vi "find_e.vi"(4 "subtract":dbl, 8 "delta thresh":dbl=2.0, 9 "square thresh":i32=2, 10 "e-size":u8, 11 "input array":dbl[][](array[numeric])) -> (3 "locations":dbl[][](array[numeric]))   [LabVIEW 2015]
uses:
  <vilib>/Analysis/_algsub.llb/Real Vector Norm.vi
  <vilib>/Analysis/baseanly.llb/Mean (DBL).vi
  <vilib>/Analysis/NI_AALPro.lvlib
  <vilib>/Analysis/NI_AALBase.lvlib
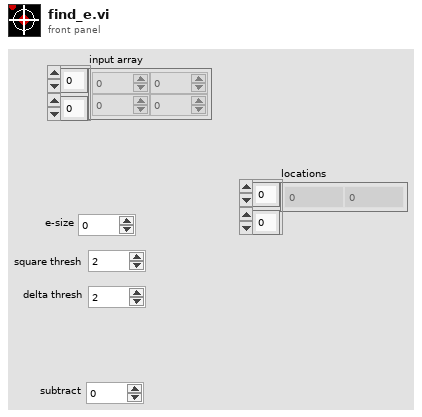
[diagram p1: front panel]
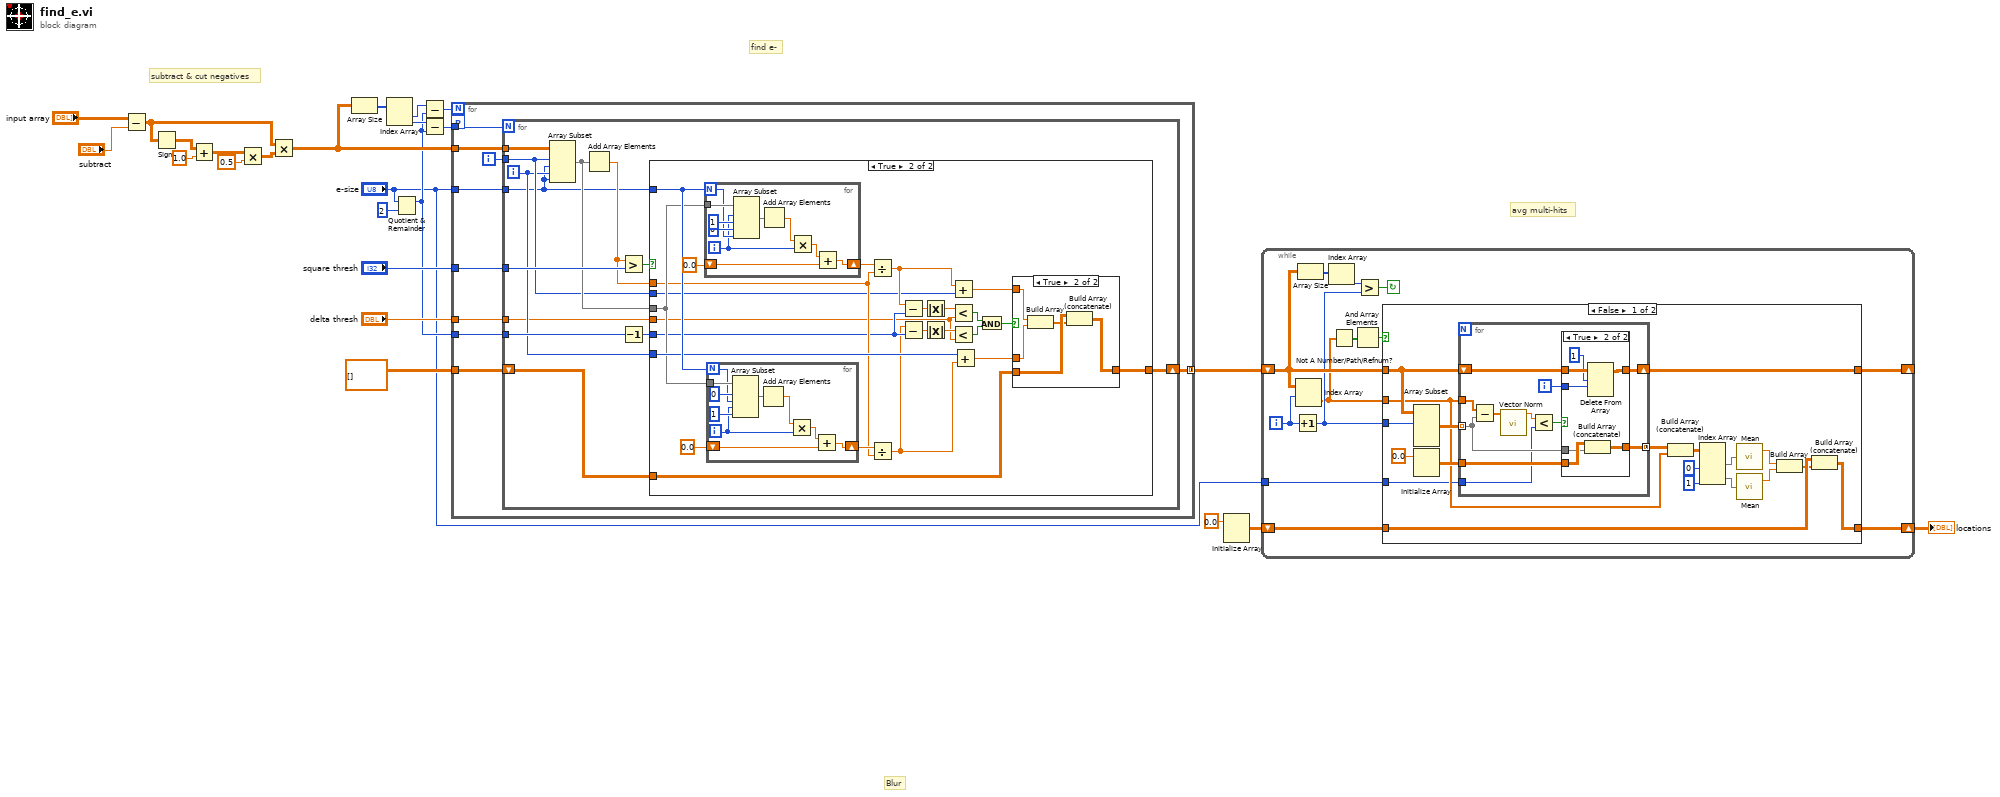
[diagram p0: block diagram]
diagram:
  # "subtract & cut negatives"
  # "avg multi-hits"
  # "find e-"
  # "Blur"
  n1 = Subtract(x="input array", y="subtract") -> (x-y=w10:dbl[][])
  n2 = Sign(1:w10) -> (0:w5:dbl[][])
  n3 = Add(x=w5, y=1.0) -> (x+y=w7:dbl[][])
  n4 = Multiply(x=w7, y=0.5) -> (x*y=w9:dbl[][])
  n5 = Multiply(x=w10, y=w9) -> (x*y=w19:dbl[][])
  n6 = Array Size(array=w19) -> (size(s)=w18:i32[])
  n7 = Index Array(array=w18) -> (element #1=w17:i32, element #2=w16:i32)  [unwired: 2 in]
  n8 = Quotient & Remainder(x="e-size", y=u8 2) -> (x-y*floor(x/y)=w3:u8)  [unwired: 1 out]
  n9 = Subtract(x=w17, y=w3) -> (x-y=w15:i32)
  n10 = Subtract(x=w16, y=w3) -> (x-y=w14:i32)
  n11 = for {
    N: w15 -> [_]
    tunnel: w19 -> [w33]
    tunnel: w14 -> [w32]
    tunnel: "e-size" -> [w30]
    tunnel: w3 -> [w29]
    tunnel: "square thresh" -> [w26]
    workers-P: _ -> [_]
    tunnel: dbl[][] [] -> [w28]
    tunnel: [w27] -> w24 mode=concatenating
    tunnel: "delta thresh" -> [w25]
    i -> [w31]
    n12 = for {
      N: w32 -> [_]
      tunnel: w33 -> [w46]
      tunnel: w31 -> [w38]
      tunnel: w30 -> [w34]
      tunnel: w29 -> [w42]
      shift-right: [w44] -> w27
      shift-left: w28 -> [w45]
      tunnel: w26 -> [w41]
      tunnel: w25 -> [w35]
      i -> [w37]
      n13 = Array Subset(array=w46, index (row)=w38, length (row)=w34, index (col)=w37, length (col)=w34) -> (w39:dbl[][])
      n14 = Add Array Elements(numeric array=w39) -> (sum=w36:dbl)
      n15 = Greater?(x=w36, y=w41) -> (0:w40:bool)
      n16 = Decrement(x=w42) -> (x-1=w43:u8)
      n17 = case shown="True" w40 {
        tunnel: w45 -> [w47 w69]
        tunnel: [w47 w68] -> w44
        tunnel: w43 -> [_ w59]
        tunnel: w34 -> [_ w67]
        tunnel: w38 -> [_ w49]
        tunnel: w37 -> [_ w64]
        tunnel: w39 -> [_ w63]
        tunnel: w36 -> [_ w60]
        tunnel: w35 -> [_ w54]
        frame False {
        }
        frame True {
          n18 = for {
            N: w67 -> [w94]
            tunnel: w63 -> [w97]
            shift-right: [w88] -> w62
            shift-left: 0.0 -> [w89]
            i -> [w91]
            n19 = Array Subset(array=w97, index (row)=w91, length (row)=1 ("Länge"), index (col)=0 ("Index"), length (col)=w94) -> (w93:dbl[][])
            n20 = Add Array Elements(numeric array=w93) -> (sum=w92:dbl)
            n21 = Multiply(x=w92, y=w91) -> (x*y=w90:dbl)
            n22 = Add(x=w90, y=w89) -> (x+y=w88:dbl)
          }
          n23 = for {
            N: w67 -> [w80]
            tunnel: w63 -> [w87]
            shift-right: [w82] -> w61
            shift-left: 0.0 -> [w83]
            i -> [w78]
            n24 = Array Subset(array=w87, index (row)=0 ("Index"), length (row)=w80, index (col)=w78, length (col)=1 ("Länge")) -> (w86:dbl[][])
            n25 = Add Array Elements(numeric array=w86) -> (sum=w85:dbl)
            n26 = Multiply(x=w85, y=w78) -> (x*y=w84:dbl)
            n27 = Add(x=w84, y=w83) -> (x+y=w82:dbl)
          }
          n28 = Divide(x=w62, y=w60) -> (x/y=w50:dbl)
          n29 = Divide(x=w61, y=w60) -> (x/y=w51:dbl)
          n30 = Subtract(x=w50, y=w59) -> (x-y=w58:dbl)
          n31 = Subtract(x=w51, y=w59) -> (x-y=w57:dbl)
          n32 = Absolute Value(x=w58) -> (abs(x)=w56:dbl)
          n33 = Absolute Value(x=w57) -> (abs(x)=w55:dbl)
          n34 = Add(x=w50, y=w49) -> (x+y=w66:dbl)
          n35 = Less?(x=w56, y=w54) -> (x < y?=w52:bool)
          n36 = Less?(x=w55, y=w54) -> (x < y?=w53:bool)
          n37 = Add(x=w64, y=w51) -> (x+y=w65:dbl)
          n38 = And(x=w52, y=w53) -> (x .and. y?=w70:bool)
          n39 = case shown="True" w70 {
            tunnel: w66 -> [_ w76]
            tunnel: w65 -> [_ w75]
            tunnel: w69 -> [w72 w77]
            tunnel: [w72 w73] -> w68
            frame False {
            }
            frame True {
              n40 = Build Array(w76, w75) -> (w74:dbl[])
              n41 = Build Array (concatenate)(w77, w74) -> (w73:dbl[][])
            }
          }
        }
      }
    }
  }
  n42 = Initialize Array(0.0 ("element")) -> (w22:dbl[][])  [unwired: 2 in]
  n43 = while {
    shift-right: [w108] -> _
    shift-left: w24 -> [w107]
    shift-right: [w109] -> w21
    shift-left: w22 -> [w110]
    tunnel: "e-size" -> [w98]
    i -> [w105]
    stop <- w102 continue-if-true
    n44 = Increment(x=w105) -> (x+1=w103:i32)
    n45 = Index Array(array=w107, index (row)=w105) -> (element=w101:dbl[])  [unwired: 1 in]
    n46 = Array Size(array=w107) -> (size(s)=w106:i32[])
    n47 = Index Array(array=w106) -> (element=w104:i32)  [unwired: 1 in]
    n48 = Not A Number/Path/Refnum?(number/path/refnum=w101) -> (NaN/Path/Refnum?=w100:bool[])
    n49 = And Array Elements(Boolean array=w100) -> (logical AND=w99:bool)
    n50 = Greater?(x=w104, y=w103) -> (0:w102:bool)
    n51 = case shown="False" w99 {
      tunnel: w110 -> [w129 w150]
      tunnel: [w128 w150] -> w109
      tunnel: [w127 w151] -> w108
      tunnel: w107 -> [w116 w151]
      tunnel: w103 -> [w115 _]
      tunnel: w101 -> [w112 _]
      tunnel: w98 -> [w111 _]
      frame False {
        n52 = Array Subset(array=w116, index (row)=w115) -> (w126:dbl[][])  [unwired: 3 in]
        n53 = Initialize Array(0.0 ("element")) -> (w124:dbl[][])  [unwired: 2 in]
        n54 = for {
          tunnel: w126 -> [w136] mode=indexing
          tunnel: w112 -> [w140]
          tunnel: w124 -> [w135]
          tunnel: [w134] -> w114 mode=concatenating
          shift-right: [w131] -> w127
          shift-left: w116 -> [w133]
          tunnel: w111 -> [w130]
          i -> [w132]
          n55 = Subtract(x=w140, y=w136) -> (x-y=w139:dbl[])
          n56 = call-poly <vilib>:"Vector Norm.vi"("Input Vector"=w139) -> ("norm"=w138:dbl)  [unwired: 9 in, 1 out]
          n57 = Less?(x=w138, y=w130) -> (x < y?=w137:bool)
          n58 = case shown="True" w137 {
            tunnel: w136 -> [_ w148]
            tunnel: w135 -> [w142 w149]
            tunnel: [w142 w147] -> w134
            tunnel: w133 -> [w141 w146]
            tunnel: w132 -> [_ w144]
            tunnel: [w141 w143] -> w131
            frame False {
            }
            frame True {
              n59 = Build Array (concatenate)(w149, w148) -> (w147:dbl[][])
              n60 = Delete From Array(array=w146, length=1, index (row)=w144) -> (array with subset deleted=w143:dbl[][])  [unwired: 1 in, 1 out]
            }
          }
        }
        n61 = Build Array (concatenate)(w114, w112) -> (w113:dbl[][])
        n62 = Index Array(array=w113, index (col) #1=0 ("disabled index (col)"), index (col) #2=1 ("index (col)")) -> (element #1=w121:dbl[], element #2=w120:dbl[])  [unwired: 2 in]
        n63 = call-poly <vilib>:"Mean.vi"("X"=w121) -> ("mean"=w119:dbl)  [unwired: 1 out]
        n64 = call-poly <vilib>:"Mean.vi"("X"=w120) -> ("mean"=w118:dbl)  [unwired: 1 out]
        n65 = Build Array(w119, w118) -> (w117:dbl[])
        n66 = Build Array (concatenate)(w129, w117) -> (w128:dbl[][])
      }
      frame True {
      }
    }
  }
  "locations" <- w21
